vi "Constructor.vi"(6 "TSP":sgl, 8 "error in":errorcluster, 9 "PID Params":cluster{"P":sgl, "I":sgl, "D":sgl}={"P"=1.0, "I"=0.75, "D"=0.0}, 10 "Ctl Params":cluster{"htx":sgl, "clx":sgl}={"htx"=0.0, "clx"=1.0}, 11 "TE Cooler in":refnum<class "TE Cooler.lvclass">) -> (0 "error out":errorcluster, 3 "TE Cooler out":refnum<class "TE Cooler.lvclass">)   [LabVIEW 2018, in "TE Cooler.lvlib" / "TE Cooler.lvclass"]
doc: "Initializes the parameters in the private part of the TEC object. This should be called before initialization or the object will be initialized with the default values."
uses:
  TE Cooler.lvclass
  TE Cooler.lvclass/TE Cooler.ctl
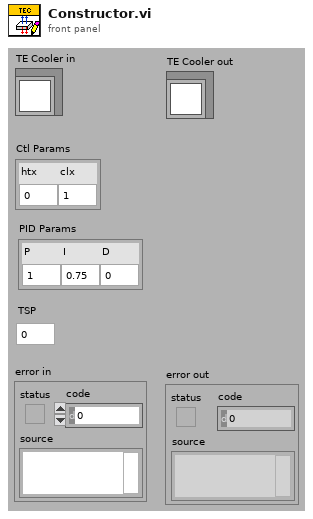
[diagram p1: front panel]
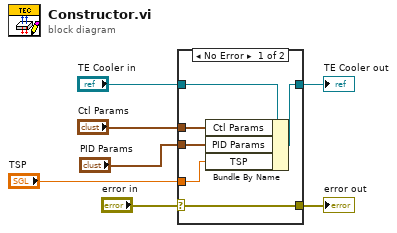
[diagram p0: block diagram]
diagram:
  n1 = case shown="No Error" "error in" {
    selector: "error in" -> [w13 w14]
    tunnel: [w13 w14] -> w6
    tunnel: [w11 w15] -> w4
    tunnel: "TE Cooler in" -> [w12 w15]
    tunnel: "Ctl Params" -> [w10 _]
    tunnel: "PID Params" -> [w9 _]
    tunnel: "TSP" -> [w8 _]
    frame No Error {
      n2 = Bundle By Name(cluster=w12, "Ctl Params"=w10, "PID Params"=w9, "TSP"=w8) -> (w11:refnum<class "TE Cooler.lvclass">)
    }
    frame Error {
    }
  }
  "error out" <- w6
  "TE Cooler out" <- w4
